vi "InitBallHandling.vi"   [LabVIEW 2020]
doc: "This VI initializes devices related directly to the intake, indexer, and tower."
uses:
  <vilib>/Rock Robotics/WPI/ThirdParty/Phoenix-LabVIEW/Motor Controller/Controls/CTRE_Phoenix_MotorControl_SupplyCurrentLimitConfiguration.ctl
  <vilib>/Rock Robotics/WPI/ThirdParty/Phoenix-LabVIEW/Motor Controller/Controls/CTRE_Phoenix_MotorControl_TalonFXInvertType.ctl
  <vilib>/Rock Robotics/WPI/ThirdParty/Phoenix-LabVIEW/Motor Controller/Controls/CTRE_Phoenix_MotorControl_NeutralMode.ctl
  <vilib>/Rock Robotics/WPI/ThirdParty/Phoenix-LabVIEW/Motor Controller/Controls/CTRE_Phoenix_MotorControl_FeedbackDevice_TalonFX.ctl
  refnumbers.vi
types:
  T1 = typedef "CTRE_Phoenix_MotorControl_FeedbackDevice_TalonFX.ctl" = i8
  T2 = typedef "CTRE_Phoenix_MotorControl_SupplyCurrentLimitConfiguration.ctl" = cluster{"Enable?":bool, "Current Limit":dbl, "Threshold Current":dbl, "Threshold Time":dbl}
  T3 = typedef "CTRE_Phoenix_MotorControl_NeutralMode.ctl" = enum8{"EEPROMSetting", "Override to Coast", "Override to Brake"}
  T4 = typedef "CTRE_Phoenix_MotorControl_TalonFXInvertType.ctl" = enum16{"Counter-Clockwise", "Clockwise"}
  T5 = typedef "WPI_MotorControlDeviceRef.ctl" = cluster{"DeviceStatus":errorcluster, "Type":T6, "PWM":cluster{"PWM Channel":T7, "DeadBand":T8}, "CAN":cluster{"Device Number":u8, "SetOutput VI Ref":variant, "GetOutput VI Ref":variant, "Enable VI Ref":variant, "Disable VI Ref":variant, "Data":variant}, "Invert":bool, "DIO PWM":cluster{"PWM \"Enable\" Channel":T7, "DIOChannel":T9, "PWM Rate":dbl}}
  T6 = typedef "WPI_MotorControlType.ctl" = enum16{"PWM", "CAN", "DIO PWM"}
  T7 = typedef "FPGA_DIOPWMChannel.ctl" = enum8{"PWM 0", "PWM 1", "PWM 2", "PWM 3", "PWM 4", "PWM 5", "PWM 6", "PWM 7", "PWM 8", "PWM 9", "PWM MXP 0", "PWM MXP 1", "PWM MXP 2", "PWM MXP 3", "PWM MXP 4", "PWM MXP 5", "PWM MXP 6", "PWM MXP 7", "PWM MXP 8", "PWM MXP 9", "Invalid"}
  T8 = typedef "WPI_PWMDeadband.ctl" = cluster{"Name":string, "maxPositivePwm":i32, "minPositivePwm":i32, "centerPwm":i32, "maxNegativePwm":i32, "minNegativePwm":i32, "angularRange":u16}
  T9 = typedef "FPGA_DIOChannel.ctl" = enum8{"DIO 0", "DIO 1", "DIO 2", "DIO 3", "DIO 4", "DIO 5", "DIO 6", "DIO 7", "DIO 8", "DIO 9", "DIO MXP 0", "DIO MXP 1", "DIO MXP 2", "DIO MXP 3", "DIO MXP 4", "DIO MXP 5", "DIO MXP 6", "DIO MXP 7", "DIO MXP 8", "DIO MXP 9", "DIO MXP 10", "DIO MXP 11", "DIO MXP 12", "DIO MXP 13", "DIO MXP 14", "DIO MXP 15", "SPI Port CS1", "SPI Port CS2", "SPI Port CS3", "SPI Port MISO", "SPI Port MOSI", "Invalid"}
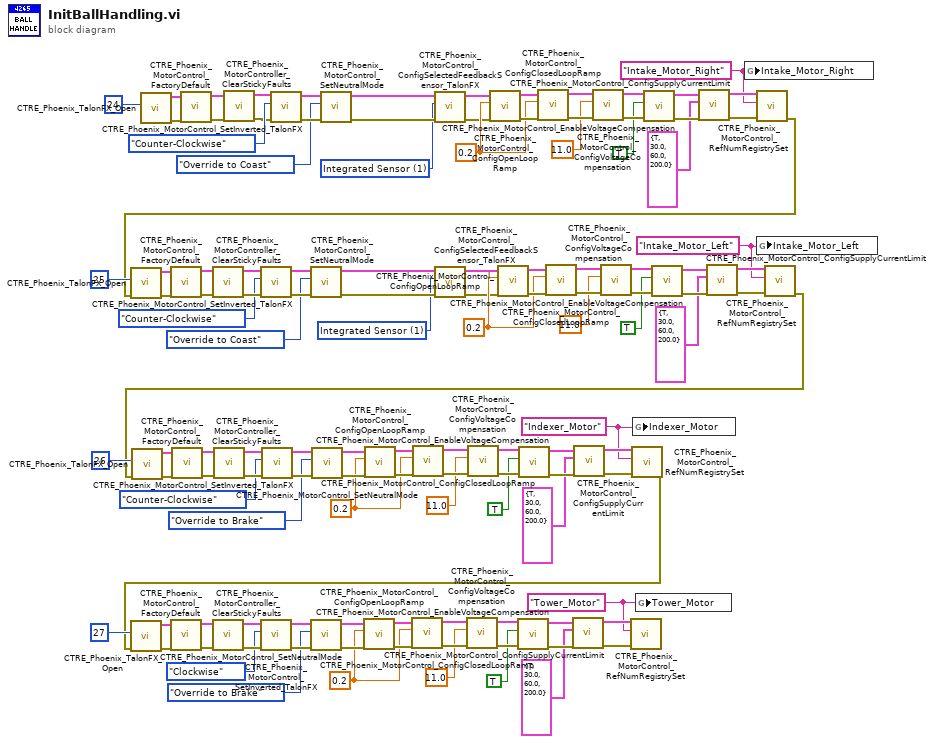
[diagram p0: block diagram]
diagram:
  w5 = T1 1 items=["Integrated Sensor"=1, "Sensor Sum (S0 + S1)"=9, "Sensor Difference (D0 - D1)"=10, "Remote Source 0"=11, "Remote Source 1"=12, "None"=14, "Software Emulated"=15] ("Talon FX Feedback Device")
  w12 = T1 1 items=["Integrated Sensor"=1, "Sensor Sum (S0 + S1)"=9, "Sensor Difference (D0 - D1)"=10, "Remote Source 0"=11, "Remote Source 1"=12, "None"=14, "Software Emulated"=15] ("Talon FX Feedback Device")
  w17 = "Intake_Motor_Right" ("refnum name")
  w29 = 0.2 ("secondsFromNeutralToFull")
  w38 = "Tower_Motor" ("refnum name")
  w52 = 0.2 ("secondsFromNeutralToFull")
  w68 = "Indexer_Motor" ("refnum name")
  w80 = 0.2 ("secondsFromNeutralToFull")
  w96 = "Intake_Motor_Left" ("refnum name")
  w108 = 0.2 ("secondsFromNeutralToFull")
  n1 = call <vilib>:"CTRE_Phoenix_TalonFX_Open.vi"("Device Number"=u8 24) -> ("error out"=w37:errorcluster, "PhoenixMotorControlDevRef"=w36:T5)  [unwired: 9 in]
  n2 = call <vilib>:"CTRE_Phoenix_MotorControl_FactoryDefault.vi"("error in"=w37, "PhoenixMotorControlDevRef"=w36) -> ("error out"=w4:errorcluster, "PhoenixMotorControlDevRef"=w3:T5)  [unwired: 8 in]
  n3 = call <vilib>:"CTRE_Phoenix_MotorController_ClearStickyFaults.vi"("error in"=w4, "PhoenixMotorControlDevRef"=w3) -> ("error out"=w1:errorcluster, "PhoenixMotorControlDevRef"=w2:T5)  [unwired: 8 in]
  n4 = call <vilib>:"CTRE_Phoenix_MotorControl_SetInverted_TalonFX.vi"("error in (no error)"=w1, "Invert Type"=CTRE_Phoenix_MotorControl_TalonFXInvertType."Counter-Clockwise", "PhoenixMotorControlDevRef"=w2) -> ("error out"=w34:errorcluster, "PhoenixMotorControlDevRef"=w33:T5)  [unwired: 7 in]
  n5 = call <vilib>:"CTRE_Phoenix_MotorControl_SetNeutralMode.vi"("error in (no error)"=w34, "Motor Control Neutral Mode"=CTRE_Phoenix_MotorControl_NeutralMode."Override to Coast", "PhoenixMotorControlDevRef"=w33) -> ("error out"=w13:errorcluster, "PhoenixMotorControlDevRef"=w14:T5)  [unwired: 7 in]
  n6 = call <vilib>:"CTRE_Phoenix_MotorControl_ConfigSelectedFeedbackSensor_TalonFX.vi"("error in (no error)"=w13, "Talon FX Feedback Device"=w12, "PhoenixMotorControlDevRef"=w14) -> ("error out"=w10:errorcluster, "PhoenixMotorControlDevRef"=w11:T5)  [unwired: 7 in]
  n7 = call <vilib>:"CTRE_Phoenix_MotorControl_ConfigOpenLoopRamp.vi"("error in (no error)"=w10, "secondsFromNeutralToFull"=w29, "PhoenixMotorControlDevRef"=w11) -> ("error out"=w31:errorcluster, "PhoenixMotorControlDevRef"=w30:T5)  [unwired: 7 in]
  n8 = call <vilib>:"CTRE_Phoenix_MotorControl_ConfigClosedLoopRamp.vi"("error in (no error)"=w31, "secondsFromNeutralToFull"=w29, "PhoenixMotorControlDevRef"=w30) -> ("error out"=w28:errorcluster, "PhoenixMotorControlDevRef"=w27:T5)  [unwired: 7 in]
  n9 = call <vilib>:"CTRE_Phoenix_MotorControl_ConfigVoltageCompensation.vi"("error in (no error)"=w28, "Saturation Voltage"=11.0, "PhoenixMotorControlDevRef"=w27) -> ("error out"=w25:errorcluster, "PhoenixMotorControlDevRef"=w24:T5)  [unwired: 7 in]
  n10 = global write "refnumbers.vi" "Indexer_Motor"(w68) -> ()
  n11 = global write "refnumbers.vi" "Tower_Motor"(w38) -> ()
  n12 = call <vilib>:"CTRE_Phoenix_MotorControl_EnableVoltageCompensation.vi"("error in (no error)"=w25, "Enable Voltage Compensation?"=TRUE, "PhoenixMotorControlDevRef"=w24) -> ("error out"=w22:errorcluster, "PhoenixMotorControlDevRef"=w21:T5)  [unwired: 7 in]
  n13 = call <vilib>:"CTRE_Phoenix_MotorControl_ConfigSupplyCurrentLimit.vi"("error in (no error)"=w22, "Supply Current Limit Configuration"=T2 {"Enable?"=TRUE, "Current Limit"=30.0, "Threshold Current"=60.0, "Threshold Time"=200.0}, "PhoenixMotorControlDevRef"=w21) -> ("error out"=w19:errorcluster, "PhoenixMotorControlDevRef"=w18:T5)  [unwired: 7 in]
  n14 = global write "refnumbers.vi" "Intake_Motor_Right"(w17) -> ()
  n15 = call <vilib>:"CTRE_Phoenix_MotorControl_RefNumRegistrySet.vi"("error in (no error)"=w19, "refnum name"=w17, "PhoenixMotorControlDevRef"=w18) -> ("error out"=w15:errorcluster)  [unwired: 7 in, 1 out]
  n16 = call <vilib>:"CTRE_Phoenix_TalonFX_Open.vi"("error in"=w15, "Device Number"=u8 25) -> ("error out"=w120:errorcluster, "PhoenixMotorControlDevRef"=w119:T5)  [unwired: 8 in]
  n17 = call <vilib>:"CTRE_Phoenix_MotorControl_FactoryDefault.vi"("error in"=w120, "PhoenixMotorControlDevRef"=w119) -> ("error out"=w118:errorcluster, "PhoenixMotorControlDevRef"=w117:T5)  [unwired: 8 in]
  n18 = call <vilib>:"CTRE_Phoenix_MotorController_ClearStickyFaults.vi"("error in"=w118, "PhoenixMotorControlDevRef"=w117) -> ("error out"=w116:errorcluster, "PhoenixMotorControlDevRef"=w115:T5)  [unwired: 8 in]
  n19 = call <vilib>:"CTRE_Phoenix_MotorControl_SetInverted_TalonFX.vi"("error in (no error)"=w116, "Invert Type"=CTRE_Phoenix_MotorControl_TalonFXInvertType."Counter-Clockwise", "PhoenixMotorControlDevRef"=w115) -> ("error out"=w113:errorcluster, "PhoenixMotorControlDevRef"=w112:T5)  [unwired: 7 in]
  n20 = call <vilib>:"CTRE_Phoenix_MotorControl_SetNeutralMode.vi"("error in (no error)"=w113, "Motor Control Neutral Mode"=CTRE_Phoenix_MotorControl_NeutralMode."Override to Coast", "PhoenixMotorControlDevRef"=w112) -> ("error out"=w8:errorcluster, "PhoenixMotorControlDevRef"=w9:T5)  [unwired: 7 in]
  n21 = call <vilib>:"CTRE_Phoenix_MotorControl_ConfigSelectedFeedbackSensor_TalonFX.vi"("error in (no error)"=w8, "Talon FX Feedback Device"=w5, "PhoenixMotorControlDevRef"=w9) -> ("error out"=w6:errorcluster, "PhoenixMotorControlDevRef"=w7:T5)  [unwired: 7 in]
  n22 = call <vilib>:"CTRE_Phoenix_MotorControl_ConfigOpenLoopRamp.vi"("error in (no error)"=w6, "secondsFromNeutralToFull"=w108, "PhoenixMotorControlDevRef"=w7) -> ("error out"=w110:errorcluster, "PhoenixMotorControlDevRef"=w109:T5)  [unwired: 7 in]
  n23 = call <vilib>:"CTRE_Phoenix_MotorControl_ConfigClosedLoopRamp.vi"("error in (no error)"=w110, "secondsFromNeutralToFull"=w108, "PhoenixMotorControlDevRef"=w109) -> ("error out"=w107:errorcluster, "PhoenixMotorControlDevRef"=w106:T5)  [unwired: 7 in]
  n24 = call <vilib>:"CTRE_Phoenix_MotorControl_ConfigVoltageCompensation.vi"("error in (no error)"=w107, "Saturation Voltage"=11.0, "PhoenixMotorControlDevRef"=w106) -> ("error out"=w104:errorcluster, "PhoenixMotorControlDevRef"=w103:T5)  [unwired: 7 in]
  n25 = call <vilib>:"CTRE_Phoenix_MotorControl_EnableVoltageCompensation.vi"("error in (no error)"=w104, "Enable Voltage Compensation?"=TRUE, "PhoenixMotorControlDevRef"=w103) -> ("error out"=w101:errorcluster, "PhoenixMotorControlDevRef"=w100:T5)  [unwired: 7 in]
  n26 = call <vilib>:"CTRE_Phoenix_MotorControl_ConfigSupplyCurrentLimit.vi"("error in (no error)"=w101, "Supply Current Limit Configuration"=T2 {"Enable?"=TRUE, "Current Limit"=30.0, "Threshold Current"=60.0, "Threshold Time"=200.0}, "PhoenixMotorControlDevRef"=w100) -> ("error out"=w98:errorcluster, "PhoenixMotorControlDevRef"=w97:T5)  [unwired: 7 in]
  n27 = global write "refnumbers.vi" "Intake_Motor_Left"(w96) -> ()
  n28 = call <vilib>:"CTRE_Phoenix_MotorControl_RefNumRegistrySet.vi"("error in (no error)"=w98, "refnum name"=w96, "PhoenixMotorControlDevRef"=w97) -> ("error out"=w40:errorcluster)  [unwired: 7 in, 1 out]
  n29 = call <vilib>:"CTRE_Phoenix_TalonFX_Open.vi"("error in"=w40, "Device Number"=u8 26) -> ("error out"=w94:errorcluster, "PhoenixMotorControlDevRef"=w93:T5)  [unwired: 8 in]
  n30 = call <vilib>:"CTRE_Phoenix_MotorControl_FactoryDefault.vi"("error in"=w94, "PhoenixMotorControlDevRef"=w93) -> ("error out"=w92:errorcluster, "PhoenixMotorControlDevRef"=w91:T5)  [unwired: 8 in]
  n31 = call <vilib>:"CTRE_Phoenix_MotorController_ClearStickyFaults.vi"("error in"=w92, "PhoenixMotorControlDevRef"=w91) -> ("error out"=w90:errorcluster, "PhoenixMotorControlDevRef"=w89:T5)  [unwired: 8 in]
  n32 = call <vilib>:"CTRE_Phoenix_MotorControl_SetInverted_TalonFX.vi"("error in (no error)"=w90, "Invert Type"=CTRE_Phoenix_MotorControl_TalonFXInvertType."Counter-Clockwise", "PhoenixMotorControlDevRef"=w89) -> ("error out"=w87:errorcluster, "PhoenixMotorControlDevRef"=w86:T5)  [unwired: 7 in]
  n33 = call <vilib>:"CTRE_Phoenix_MotorControl_SetNeutralMode.vi"("error in (no error)"=w87, "Motor Control Neutral Mode"=CTRE_Phoenix_MotorControl_NeutralMode."Override to Brake", "PhoenixMotorControlDevRef"=w86) -> ("error out"=w84:errorcluster, "PhoenixMotorControlDevRef"=w83:T5)  [unwired: 7 in]
  n34 = call <vilib>:"CTRE_Phoenix_MotorControl_ConfigOpenLoopRamp.vi"("error in (no error)"=w84, "secondsFromNeutralToFull"=w80, "PhoenixMotorControlDevRef"=w83) -> ("error out"=w82:errorcluster, "PhoenixMotorControlDevRef"=w81:T5)  [unwired: 7 in]
  n35 = call <vilib>:"CTRE_Phoenix_MotorControl_ConfigClosedLoopRamp.vi"("error in (no error)"=w82, "secondsFromNeutralToFull"=w80, "PhoenixMotorControlDevRef"=w81) -> ("error out"=w79:errorcluster, "PhoenixMotorControlDevRef"=w78:T5)  [unwired: 7 in]
  n36 = call <vilib>:"CTRE_Phoenix_MotorControl_ConfigVoltageCompensation.vi"("error in (no error)"=w79, "Saturation Voltage"=11.0, "PhoenixMotorControlDevRef"=w78) -> ("error out"=w76:errorcluster, "PhoenixMotorControlDevRef"=w75:T5)  [unwired: 7 in]
  n37 = call <vilib>:"CTRE_Phoenix_MotorControl_EnableVoltageCompensation.vi"("error in (no error)"=w76, "Enable Voltage Compensation?"=TRUE, "PhoenixMotorControlDevRef"=w75) -> ("error out"=w73:errorcluster, "PhoenixMotorControlDevRef"=w72:T5)  [unwired: 7 in]
  n38 = call <vilib>:"CTRE_Phoenix_MotorControl_ConfigSupplyCurrentLimit.vi"("error in (no error)"=w73, "Supply Current Limit Configuration"=T2 {"Enable?"=TRUE, "Current Limit"=30.0, "Threshold Current"=60.0, "Threshold Time"=200.0}, "PhoenixMotorControlDevRef"=w72) -> ("error out"=w70:errorcluster, "PhoenixMotorControlDevRef"=w69:T5)  [unwired: 7 in]
  n39 = call <vilib>:"CTRE_Phoenix_MotorControl_RefNumRegistrySet.vi"("error in (no error)"=w70, "refnum name"=w68, "PhoenixMotorControlDevRef"=w69) -> ("error out"=w39:errorcluster)  [unwired: 7 in, 1 out]
  n40 = call <vilib>:"CTRE_Phoenix_TalonFX_Open.vi"("error in"=w39, "Device Number"=u8 27) -> ("error out"=w66:errorcluster, "PhoenixMotorControlDevRef"=w65:T5)  [unwired: 8 in]
  n41 = call <vilib>:"CTRE_Phoenix_MotorControl_FactoryDefault.vi"("error in"=w66, "PhoenixMotorControlDevRef"=w65) -> ("error out"=w64:errorcluster, "PhoenixMotorControlDevRef"=w63:T5)  [unwired: 8 in]
  n42 = call <vilib>:"CTRE_Phoenix_MotorController_ClearStickyFaults.vi"("error in"=w64, "PhoenixMotorControlDevRef"=w63) -> ("error out"=w62:errorcluster, "PhoenixMotorControlDevRef"=w61:T5)  [unwired: 8 in]
  n43 = call <vilib>:"CTRE_Phoenix_MotorControl_SetInverted_TalonFX.vi"("error in (no error)"=w62, "Invert Type"=CTRE_Phoenix_MotorControl_TalonFXInvertType."Clockwise", "PhoenixMotorControlDevRef"=w61) -> ("error out"=w59:errorcluster, "PhoenixMotorControlDevRef"=w58:T5)  [unwired: 7 in]
  n44 = call <vilib>:"CTRE_Phoenix_MotorControl_SetNeutralMode.vi"("error in (no error)"=w59, "Motor Control Neutral Mode"=CTRE_Phoenix_MotorControl_NeutralMode."Override to Brake", "PhoenixMotorControlDevRef"=w58) -> ("error out"=w56:errorcluster, "PhoenixMotorControlDevRef"=w55:T5)  [unwired: 7 in]
  n45 = call <vilib>:"CTRE_Phoenix_MotorControl_ConfigOpenLoopRamp.vi"("error in (no error)"=w56, "secondsFromNeutralToFull"=w52, "PhoenixMotorControlDevRef"=w55) -> ("error out"=w54:errorcluster, "PhoenixMotorControlDevRef"=w53:T5)  [unwired: 7 in]
  n46 = call <vilib>:"CTRE_Phoenix_MotorControl_ConfigClosedLoopRamp.vi"("error in (no error)"=w54, "secondsFromNeutralToFull"=w52, "PhoenixMotorControlDevRef"=w53) -> ("error out"=w51:errorcluster, "PhoenixMotorControlDevRef"=w50:T5)  [unwired: 7 in]
  n47 = call <vilib>:"CTRE_Phoenix_MotorControl_ConfigVoltageCompensation.vi"("error in (no error)"=w51, "Saturation Voltage"=11.0, "PhoenixMotorControlDevRef"=w50) -> ("error out"=w48:errorcluster, "PhoenixMotorControlDevRef"=w47:T5)  [unwired: 7 in]
  n48 = call <vilib>:"CTRE_Phoenix_MotorControl_EnableVoltageCompensation.vi"("error in (no error)"=w48, "Enable Voltage Compensation?"=TRUE, "PhoenixMotorControlDevRef"=w47) -> ("error out"=w45:errorcluster, "PhoenixMotorControlDevRef"=w44:T5)  [unwired: 7 in]
  n49 = call <vilib>:"CTRE_Phoenix_MotorControl_ConfigSupplyCurrentLimit.vi"("error in (no error)"=w45, "Supply Current Limit Configuration"=T2 {"Enable?"=TRUE, "Current Limit"=30.0, "Threshold Current"=60.0, "Threshold Time"=200.0}, "PhoenixMotorControlDevRef"=w44) -> ("error out"=w42:errorcluster, "PhoenixMotorControlDevRef"=w41:T5)  [unwired: 7 in]
  n50 = call <vilib>:"CTRE_Phoenix_MotorControl_RefNumRegistrySet.vi"("error in (no error)"=w42, "refnum name"=w38, "PhoenixMotorControlDevRef"=w41) -> ()  [unwired: 7 in, 2 out]
